vi "Count.vi"(8 "error in (no error)":errorcluster, 11 "StringList in":refnum<class "StringList.lvclass">) -> (0 "error out":errorcluster, 2 "Number of Items":i32, 3 "StringList out":refnum<class "StringList.lvclass">)   [LabVIEW 2017, in "LapDog.Collections.v0.Lists.Interfaces.lvlib" / "StringList.lvclass"]
uses:
  StringList.lvclass
  StringList.lvclass/StringList.ctl
  Lists/List/List.lvclass
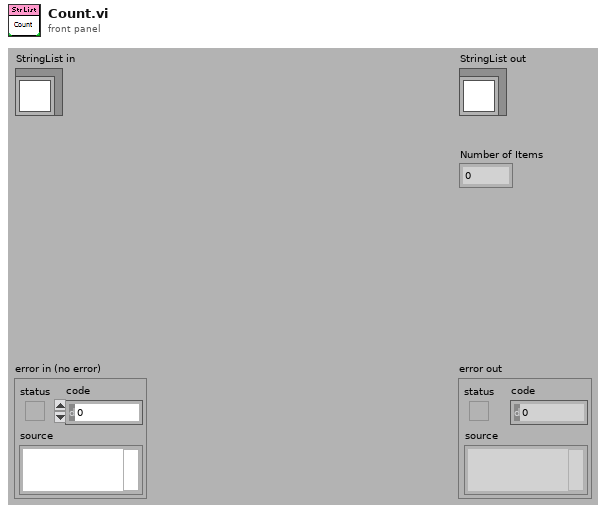
[diagram p1: front panel]
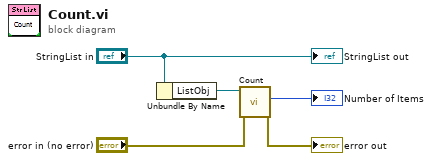
[diagram p0: block diagram]
diagram:
  n1 = Unbundle By Name("StringList in") -> ("ListObj"=w4:refnum<class "List.lvclass">)
  n2 = call-dynamic "Count.vi"("error in (no error)"="error in (no error)", "List in"=w4) -> ("error out"=→"error out":errorcluster, "Number of Items"=→"Number of Items":i32)  [unwired: 7 in, 1 out]
  "StringList out" <- "StringList in"
